vi "Priority system.vi"(0 "robot location":dbl[](array[numeric]), 1 "robot direction":string, 3 "Display Map":dbl[][](array[numeric])) -> (7 "Map":u16[][](array[ring]), 8 "target location":dbl[](array[numeric]))   [LabVIEW 2015]
uses:
  <vilib>/robotics/Navigation/shared/WorldMap/OccupancyGridWorldMap/NI_Robotics_OccupancyGridWorldMap.lvclass
  <vilib>/robotics/Navigation/NI_Robotics_Navigation .lvlib
panel:
  out "route map":dbl[][](array[numeric])
  out "distances":dbl[](array[numeric])
  out "Indices":i32[][](array[numeric])
  out "Priority level array":dbl[][](array[numeric])
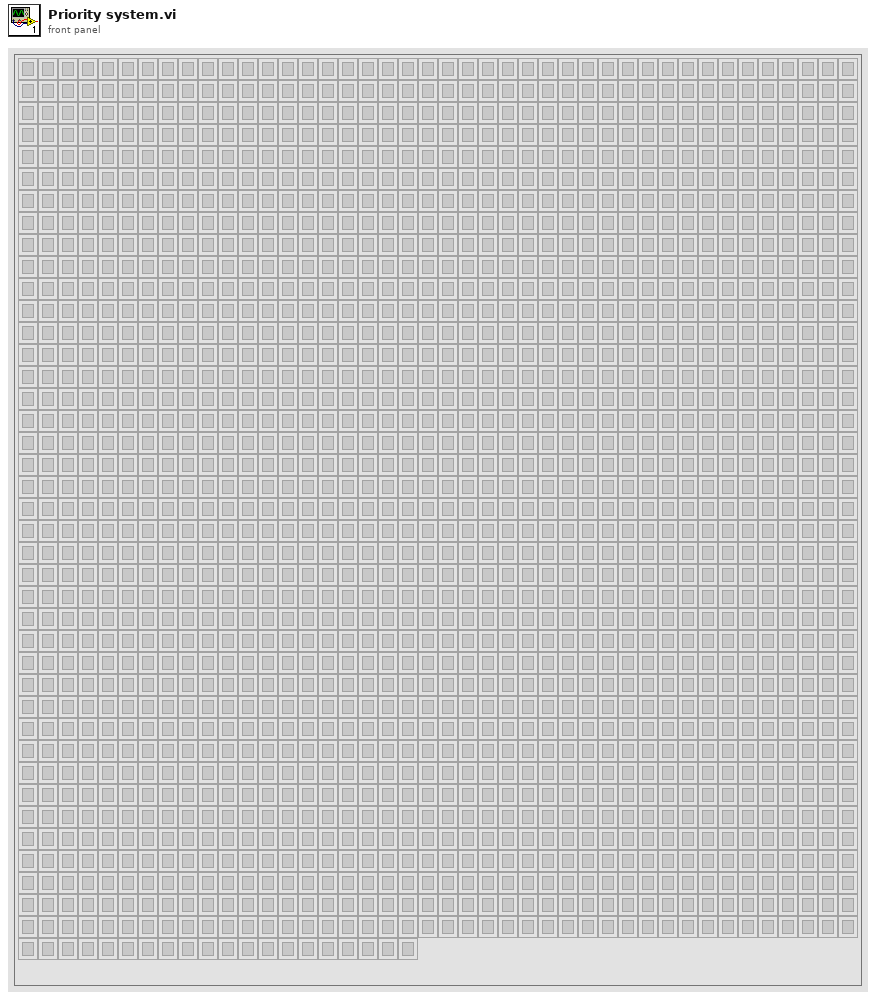
[diagram p1: front panel]
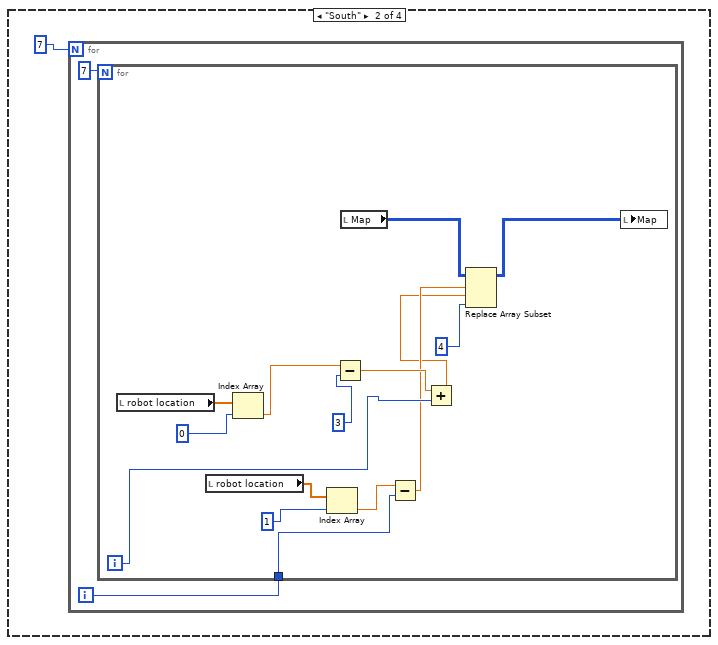
[diagram p2: hidden frame]
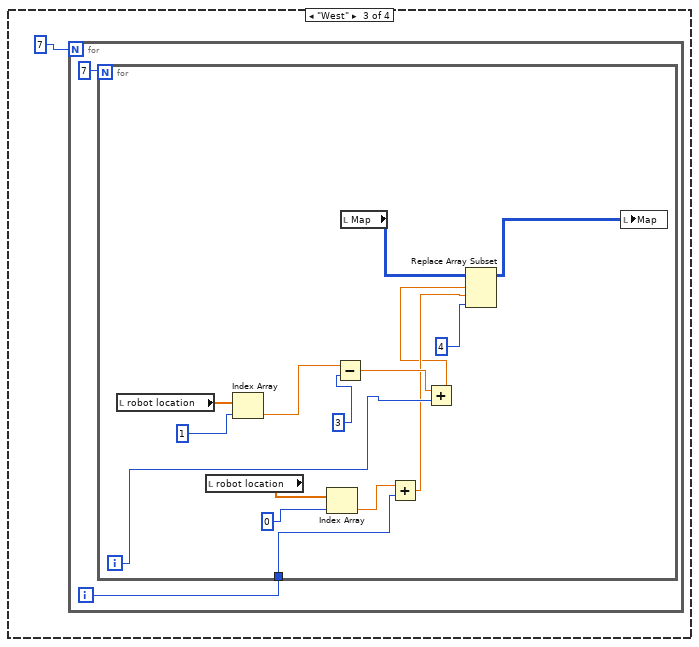
[diagram p3: hidden frame]
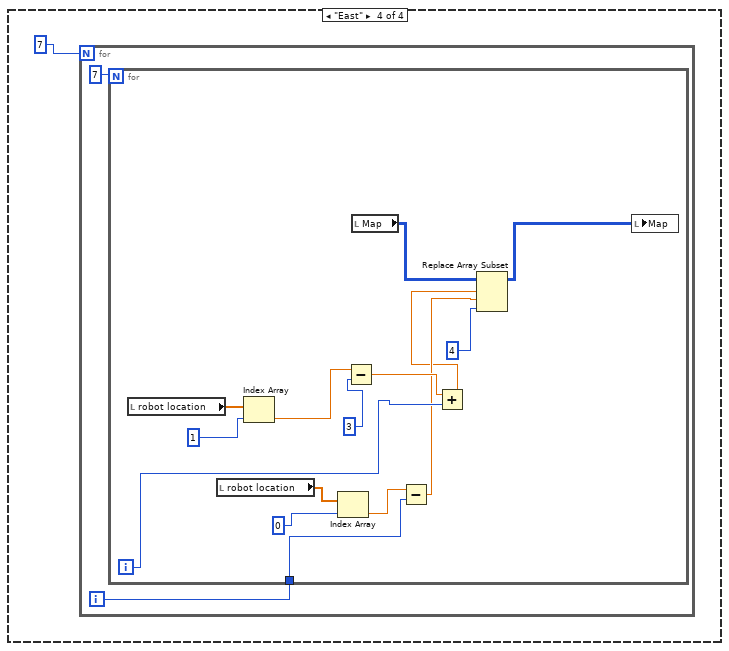
[diagram p4: hidden frame]
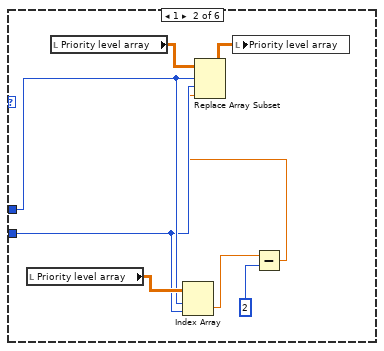
[diagram p6: hidden frame]
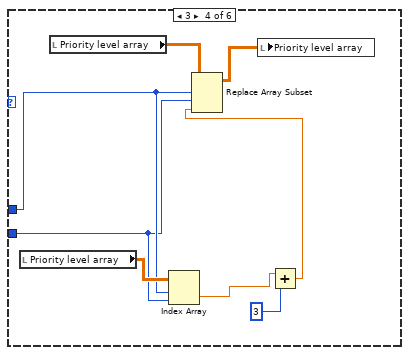
[diagram p8: hidden frame]
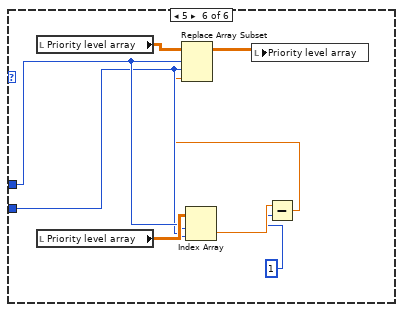
[diagram p9: hidden frame]
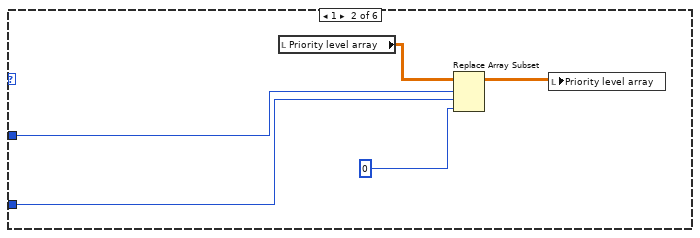
[diagram p10: hidden frame]
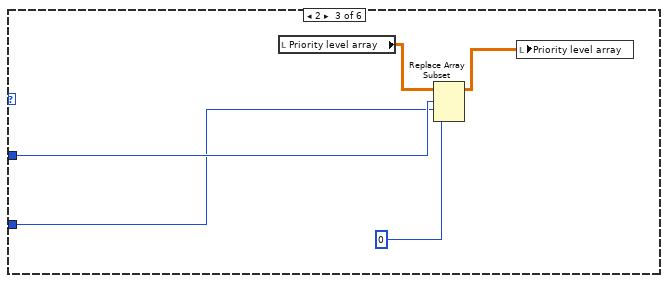
[diagram p11: hidden frame]
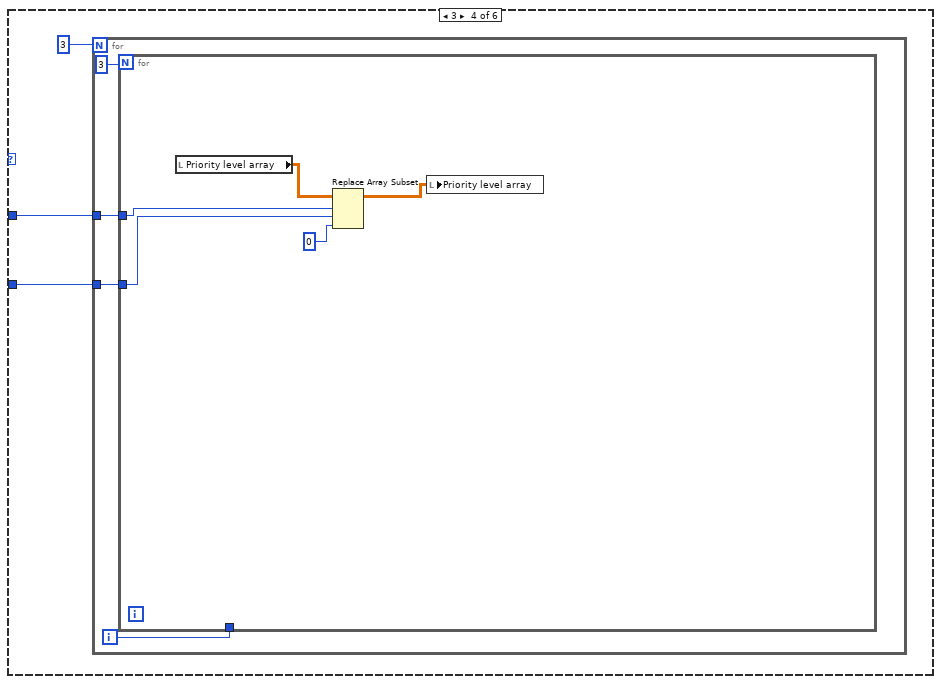
[diagram p12: hidden frame]
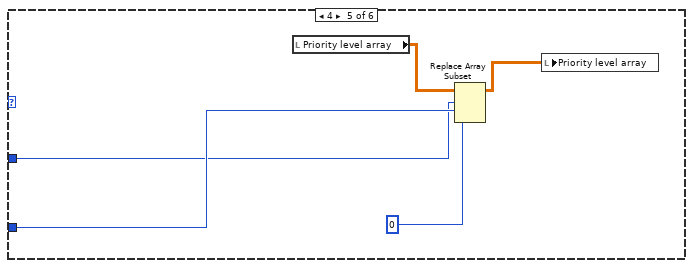
[diagram p13: hidden frame]
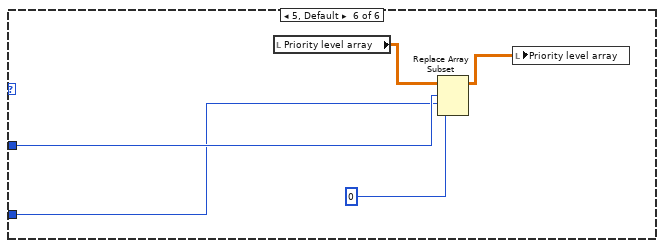
[diagram p14: hidden frame]
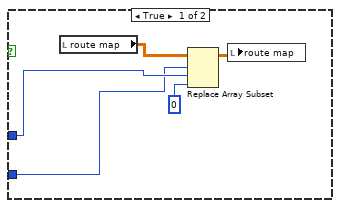
[diagram p16: hidden frame]
diagram:
  n1 = flat-sequence {
    frame #0 {
      "Map" <- "Display Map"
      "Priority level array" <- "Display Map"
      "route map" <- "Display Map"
    }
    frame #1 {
      n2 = for {
        N: 40 -> [_]
        i -> [w3]
        n3 = for {
          N: 40 -> [_]
          tunnel: w3 -> [w9]
          i -> [w10]
          n4 = local read "Priority level array"() -> (w5:dbl[][])
          n5 = local read "route map"() -> (w6:dbl[][])
          n6 = Replace Array Subset(array=w6, new element=0, index (row)=w10, index (col)=w9) -> (w11:dbl[][])
          n7 = Replace Array Subset(array=w5, new element=15, index (row)=w10, index (col)=w9) -> (w12:dbl[][])
          n8 = local write "Priority level array"(w12) -> ()
          n9 = local write "route map"(w11) -> ()
        }
      }
    }
    frame #2 {
      n10 = case shown="\"North\", Default" "robot direction" {
        frame "North", Default {
          n11 = for {
            N: 7 -> [_]
            i -> [w15]
            n12 = for {
              N: 7 -> [_]
              tunnel: w15 -> [w23]
              i -> [w27]
              n13 = local read "robot location"() -> (w17:dbl[])
              n14 = local read "robot location"() -> (w20:dbl[])
              n15 = Index Array(array=w17, index=0) -> (element=w18:dbl)
              n16 = Index Array(array=w20, index=1) -> (element=w19:dbl)
              n17 = Subtract(x=w18, y=3) -> (x-y=w26:dbl)
              n18 = local read "Map"() -> (w22:u16[][])
              n19 = Add(x=w19, y=w23) -> (x+y=w25:dbl)
              n20 = Add(x=w26, y=w27) -> (x+y=w24:dbl)
              n21 = Replace Array Subset(array=w22, new element=4, index (row)=w25, index (col)=w24) -> (w21:u16[][])
              n22 = local write "Map"(w21) -> ()
            }
          }
        }
        frame "South" {
          n23 = for {
            N: 7 -> [_]
            i -> [w33]
            n24 = for {
              N: 7 -> [_]
              tunnel: w33 -> [w41]
              i -> [w45]
              n25 = local read "robot location"() -> (w38:dbl[])
              n26 = local read "robot location"() -> (w37:dbl[])
              n27 = Index Array(array=w38, index=0) -> (element=w36:dbl)
              n28 = Index Array(array=w37, index=1) -> (element=w35:dbl)
              n29 = Subtract(x=w36, y=3) -> (x-y=w44:dbl)
              n30 = local read "Map"() -> (w40:u16[][])
              n31 = Subtract(x=w35, y=w41) -> (x-y=w43:dbl)
              n32 = Add(x=w44, y=w45) -> (x+y=w42:dbl)
              n33 = Replace Array Subset(array=w40, new element=4, index (row)=w43, index (col)=w42) -> (w39:u16[][])
              n34 = local write "Map"(w39) -> ()
            }
          }
        }
        frame "West" {
          n35 = for {
            N: 7 -> [_]
            i -> [w51]
            n36 = for {
              N: 7 -> [_]
              tunnel: w51 -> [w61]
              i -> [w63]
              n37 = local read "robot location"() -> (w56:dbl[])
              n38 = local read "robot location"() -> (w55:dbl[])
              n39 = Index Array(array=w56, index=1) -> (element=w54:dbl)
              n40 = Index Array(array=w55, index=0) -> (element=w53:dbl)
              n41 = Subtract(x=w54, y=3) -> (x-y=w62:dbl)
              n42 = local read "Map"() -> (w58:u16[][])
              n43 = Add(x=w53, y=w61) -> (x+y=w60:dbl)
              n44 = Add(x=w62, y=w63) -> (x+y=w59:dbl)
              n45 = Replace Array Subset(array=w58, new element=4, index (row)=w59, index (col)=w60) -> (w57:u16[][])
              n46 = local write "Map"(w57) -> ()
            }
          }
        }
        frame "East" {
          n47 = for {
            N: 7 -> [_]
            i -> [w69]
            n48 = for {
              N: 7 -> [_]
              tunnel: w69 -> [w73]
              i -> [w75]
              n49 = local read "robot location"() -> (w82:dbl[])
              n50 = local read "robot location"() -> (w80:dbl[])
              n51 = Index Array(array=w82, index=1) -> (element=w77:dbl)
              n52 = Index Array(array=w80, index=0) -> (element=w78:dbl)
              n53 = Subtract(x=w77, y=3) -> (x-y=w74:dbl)
              n54 = local read "Map"() -> (w85:u16[][])
              n55 = Subtract(x=w78, y=w73) -> (x-y=w72:dbl)
              n56 = Add(x=w74, y=w75) -> (x+y=w71:dbl)
              n57 = Replace Array Subset(array=w85, new element=4, index (row)=w71, index (col)=w72) -> (w84:u16[][])
              n58 = local write "Map"(w84) -> ()
            }
          }
        }
      }
    }
    frame #3 {
    }
    frame #4 {
      n59 = for {
        N: 40 -> [_]
        i -> [w87]
        n60 = for {
          N: 40 -> [_]
          tunnel: w87 -> [w91]
          i -> [w90]
          n61 = local read "Map"() -> (w92:u16[][])
          n62 = Index Array(array=w92, index (row)=w90, index (col)=w91) -> (element=w89:u16)
          n63 = case shown="0" w89 {
            tunnel: w91 -> [w95 w145 w151 w156 w168 w172]
            tunnel: w90 -> [w94 w144 w152 w155 w167 w173]
            frame 0 {
              n64 = for {
                N: 3 -> [_]
                tunnel: w95 -> [w99]
                tunnel: w94 -> [w98]
                i -> [w96]
                n65 = for {
                  N: 3 -> [_]
                  tunnel: w99 -> [w108]
                  tunnel: w98 -> [w107]
                  tunnel: w96 -> [w103]
                  i -> [w105]
                  n66 = Add(x=w107, y=1) -> (x+y=w106:i32)
                  n67 = Add(x=w108, y=1) -> (x+y=w104:i32)
                  n68 = local read "Map"() -> (w111:u16[][])
                  n69 = Subtract(x=w106, y=w105) -> (x-y=w101:i32)
                  n70 = Subtract(x=w104, y=w103) -> (x-y=w102:i32)
                  n71 = Index Array(array=w111, index (row)=w101, index (col)=w102) -> (element=w100:u16)
                  n72 = case shown="4" w100 {
                    tunnel: w108 -> [_ w115 _ w124 w131 w139]
                    tunnel: w107 -> [_ w116 _ w125 w132 w140]
                    frame 0, Default {
                    }
                    frame 1 {
                      n73 = local read "Priority level array"() -> (w119:dbl[][])
                      n74 = local read "Priority level array"() -> (w118:dbl[][])
                      n75 = Index Array(array=w119, index (row)=w116, index (col)=w115) -> (element=w114:dbl)
                      n76 = Subtract(x=w114, y=2) -> (x-y=w112:dbl)
                      n77 = Replace Array Subset(array=w118, new element=w112, index (row)=w116, index (col)=w115) -> (w117:dbl[][])
                      n78 = local write "Priority level array"(w117) -> ()
                    }
                    frame 2 {
                    }
                    frame 3 {
                      n79 = local read "Priority level array"() -> (w126:dbl[][])
                      n80 = local read "Priority level array"() -> (w127:dbl[][])
                      n81 = Index Array(array=w126, index (row)=w125, index (col)=w124) -> (element=w123:dbl)
                      n82 = Add(x=w123, y=3) -> (x+y=w121:dbl)
                      n83 = Replace Array Subset(array=w127, new element=w121, index (row)=w125, index (col)=w124) -> (w122:dbl[][])
                      n84 = local write "Priority level array"(w122) -> ()
                    }
                    frame 4 {
                      n85 = local read "Priority level array"() -> (w133:dbl[][])
                      n86 = local read "Priority level array"() -> (w135:dbl[][])
                      n87 = Index Array(array=w133, index (row)=w132, index (col)=w131) -> (element=w130:dbl)
                      n88 = Subtract(x=w130, y=0) -> (x-y=w129:dbl)
                      n89 = Replace Array Subset(array=w135, new element=w129, index (row)=w132, index (col)=w131) -> (w134:dbl[][])
                      n90 = local write "Priority level array"(w134) -> ()
                    }
                    frame 5 {
                      n91 = local read "Priority level array"() -> (w141:dbl[][])
                      n92 = local read "Priority level array"() -> (w143:dbl[][])
                      n93 = Index Array(array=w143, index (row)=w140, index (col)=w139) -> (element=w138:dbl)
                      n94 = Subtract(x=w138, y=1) -> (x-y=w137:dbl)
                      n95 = Replace Array Subset(array=w141, new element=w137, index (row)=w140, index (col)=w139) -> (w142:dbl[][])
                      n96 = local write "Priority level array"(w142) -> ()
                    }
                  }
                }
              }
            }
            frame 1 {
              n97 = local read "Priority level array"() -> (w148:dbl[][])
              n98 = Replace Array Subset(array=w148, new element=0, index (row)=w144, index (col)=w145) -> (w147:dbl[][])
              n99 = local write "Priority level array"(w147) -> ()
            }
            frame 2 {
              n100 = local read "Priority level array"() -> (w153:dbl[][])
              n101 = Replace Array Subset(array=w153, new element=0, index (row)=w152, index (col)=w151) -> (w150:dbl[][])
              n102 = local write "Priority level array"(w150) -> ()
            }
            frame 3 {
              n103 = for {
                N: 3 -> [_]
                tunnel: w156 -> [w160]
                tunnel: w155 -> [w159]
                i -> [w157]
                n104 = for {
                  N: 3 -> [_]
                  tunnel: w160 -> [w161]
                  tunnel: w159 -> [w162]
                  tunnel: w157 -> [_]
                  n105 = local read "Priority level array"() -> (w165:dbl[][])
                  n106 = Replace Array Subset(array=w165, new element=0, index (row)=w162, index (col)=w161) -> (w164:dbl[][])
                  n107 = local write "Priority level array"(w164) -> ()
                }
              }
            }
            frame 4 {
              n108 = local read "Priority level array"() -> (w170:dbl[][])
              n109 = Replace Array Subset(array=w170, new element=0, index (row)=w167, index (col)=w168) -> (w169:dbl[][])
              n110 = local write "Priority level array"(w169) -> ()
            }
            frame 5, Default {
              n111 = local read "Priority level array"() -> (w175:dbl[][])
              n112 = Replace Array Subset(array=w175, new element=0, index (row)=w173, index (col)=w172) -> (w174:dbl[][])
              n113 = local write "Priority level array"(w174) -> ()
            }
          }
        }
      }
    }
    frame #5 {
      n114 = local read "Priority level array"() -> (w177:dbl[][])
      n115 = for {
        tunnel: [w180] -> _ mode=indexing
        shift-right: [w184] -> w179
        shift-left: i32[][] [] -> [w182]
        tunnel: w177 -> [w180] mode=indexing
        i -> [w186]
        n116 = Increment(x=w186) -> (x+1=w185:i32)
        n117 = for {
          tunnel: w180 -> [w195] mode=indexing
          tunnel: w185 -> [w191]
          shift-right: [w190] -> w183
          shift-left: i32[][] [] -> [w189]
          i -> [w193]
          n118 = local read "Priority level array"() -> (w188:dbl[][])
          n119 = Array Max & Min(array=w188) -> (max value=w187:dbl)  [unwired: 3 out]
          n120 = Equal?(x=w195, y=w187) -> (x = y?=w194:bool)
          n121 = Increment(x=w193) -> (x+1=w192:i32)
          n122 = case shown="True" w194 {
            tunnel: w192 -> [_ w201]
            tunnel: w191 -> [_ w200]
            tunnel: [w196 w198] -> w190
            tunnel: w189 -> [w196 w197]
            frame False {
            }
            frame True {
              n123 = Build Array(w201, w200) -> (w199:i32[])
              n124 = Build Array (concatenate)(w197, w199) -> (w198:i32[][])
            }
          }
        }
        n125 = Build Array (concatenate)(w182, w183) -> (w184:i32[][])
      }
      "Indices" <- w179
      "distances" <- i32[] [0, 0, 0, 0]
    }
    frame #6 {
      n126 = for {
        N: 10 -> [_]
        i -> [w204]
        n127 = local read "Indices"() -> (w226:i32[][])
        n128 = Index Array(array=w226, index (row)=w204, index (col)=0) -> (element=w218:i32)
        n129 = Index Array(array=w226, index (row)=w204, index (col)=1) -> (element=w217:i32)
        n130 = Index Array(array="robot location", index=1) -> (element=w220:dbl)
        n131 = Index Array(array="robot location", index=0) -> (element=w222:dbl)
        n132 = Add(x=w220, y=1) -> (x+y=w215:dbl)
        n133 = Add(x=w222, y=1) -> (x+y=w216:dbl)
        n134 = Subtract(x=w218, y=w216) -> (x-y=w214:dbl)
        n135 = Subtract(x=w217, y=w215) -> (x-y=w207:dbl)
        n136 = Square(x=w207) -> (x^2=w213:dbl)
        n137 = Square(x=w214) -> (x^2=w212:dbl)
        n138 = Add(x=w212, y=w213) -> (x+y=w211:dbl)
        n139 = local read "distances"() -> (w210:dbl[])
        n140 = Square Root(x=w211) -> (sqrt(x)=w208:dbl)
        n141 = Replace Array Subset(array=w210, new element=w208, index=w204) -> (w209:dbl[])
        n142 = local write "distances"(w209) -> ()
      }
      "target location" <- i32[] [0, 0]
    }
    frame #7 {
      n143 = local read "distances"() -> (w234:dbl[])
      n144 = local read "Indices"() -> (w227:i32[][])
      n145 = Array Max & Min(array=w234) -> (min index (indices)=w229:i32)  [unwired: 3 out]
      n146 = local read "target location"() -> (w231:dbl[])
      n147 = Index Array(array=w227, index (row)=w229, index (col)=0) -> (element=w232:i32)
      n148 = Replace Array Subset(array=w231, new element=w232, index=0) -> (w233:dbl[])
      n149 = local write "target location"(w233) -> ()
    }
    frame #8 {
      n150 = local read "distances"() -> (w241:dbl[])
      n151 = local read "Indices"() -> (w240:i32[][])
      n152 = Array Max & Min(array=w241) -> (min index (indices)=w242:i32)  [unwired: 3 out]
      n153 = local read "target location"() -> (w237:dbl[])
      n154 = Index Array(array=w240, index (row)=w242, index (col)=1) -> (element=w236:i32)
      n155 = Replace Array Subset(array=w237, new element=w236, index=1) -> (w235:dbl[])
      n156 = local write "target location"(w235) -> ()
    }
    frame #9 {
      n157 = local read "target location"() -> (w249:dbl[])
      n158 = Index Array(array=w249, index #1=0, index #2=1) -> (element #1=w246:dbl, element #2=w245:dbl)
      n159 = local read "Map"() -> (w252:u16[][])
      n160 = Decrement(x=w245) -> (x-1=w244:dbl)
      n161 = Decrement(x=w246) -> (x-1=w243:dbl)
      n162 = Replace Array Subset(array=w252, new element=4, index (row)=w244, index (col)=w243) -> (w251:u16[][])
      n163 = local write "Map"(w251) -> ()
    }
    frame #10 {
      n164 = for {
        N: 40 -> [_]
        i -> [w254]
        n165 = for {
          N: 40 -> [_]
          tunnel: w254 -> [w259]
          i -> [w260]
          n166 = local read "Priority level array"() -> (w261:dbl[][])
          n167 = Index Array(array=w261, index (row)=w260, index (col)=w259) -> (element=w257:dbl)
          n168 = Equal?(x=w257, y=15) -> (x = y?=w258:bool)
          n169 = case shown="False" w258 {
            tunnel: w260 -> [w262 w268]
            tunnel: w259 -> [w263 w267]
            frame True {
              n170 = local read "route map"() -> (w265:dbl[][])
              n171 = Replace Array Subset(array=w265, new element=0, index (row)=w262, index (col)=w263) -> (w266:dbl[][])
              n172 = local write "route map"(w266) -> ()
            }
            frame False {
              n173 = local read "route map"() -> (w270:dbl[][])
              n174 = Replace Array Subset(array=w270, new element=1, index (row)=w268, index (col)=w267) -> (w269:dbl[][])
              n175 = local write "route map"(w269) -> ()
            }
          }
        }
      }
    }
    frame #11 {
      n176 = local read "route map"() -> (w284:dbl[][])
      n177 = local read "robot location"() -> (w283:dbl[])
      n178 = Multiply(x=w284, y=99) -> (x*y=w295:dbl[][])
      n179 = Add(x=w295, y=1) -> (x+y=w293:dbl[][])
      n180 = call <vilib>:"Create Occupancy Grid Map.vi"("occupancy grid"=w293) -> ("error out"=w292:errorcluster, "map reference out"=w288:refnum<data-value>)  [unwired: 9 in]
      n181 = Index Array(array=w283, index #1=0, index #2=1) -> (element #1=w273:dbl, element #2=w272:dbl)
      n182 = local read "target location"() -> (w280:dbl[])
      n183 = call <vilib>:"Get Cell Reference.vi"("error in (no error)"=w292, "y"=w273, "x"=w272, "map reference in"=w288) -> ("error out"=w291:errorcluster, "cell reference"=w289:refnum<data-value>, "map reference out"=w301:refnum<data-value>)  [unwired: 4 in, 1 out]
      n184 = Index Array(array=w280, index #1=0, index #2=1) -> (element #1=w277:dbl, element #2=w276:dbl)
      n185 = Decrement(x=w276) -> (x-1=w274:dbl)
      n186 = Decrement(x=w277) -> (x-1=w275:dbl)
      n187 = call <vilib>:"Get Cell Reference.vi"("error in (no error)"=w291, "y"=w275, "x"=w274, "map reference in"=w301) -> ("error out"=w290:errorcluster, "cell reference"=w287:refnum<data-value>, "map reference out"=w299:refnum<data-value>)  [unwired: 4 in, 1 out]
      n188 = call <vilib>:"A Star Plan.vi"("goal reference"=w287, "start reference"=w289, "map reference in"=w299) -> ("path references"=w300:refnum<data-value>[])  [unwired: 5 in, 3 out]
      n189 = call <vilib>:"Get Cells in Path.vi"("error in (no error)"=w290, "path references"=w300, "map reference in"=w299) -> ("error out"=w285:errorcluster, "y coordinates"=w298:i32[], "x coordinates"=w297:i32[], "map reference out"=w286:refnum<data-value>)  [unwired: 5 in]
      n190 = for {
        tunnel: w298 -> [w305] mode=indexing
        tunnel: w297 -> [w306] mode=indexing
        n191 = local read "Map"() -> (w302:u16[][])
        n192 = Replace Array Subset(array=w302, new element=2, index (row)=w306, index (col)=w305) -> (w303:u16[][])
        n193 = local write "Map"(w303) -> ()
      }
      n194 = call <vilib>:"Close Occupancy Grid Map.vi"("error in (no error)"=w285, "map reference in"=w286) -> ()  [unwired: 9 in, 1 out]
    }
    frame #12 {
      n195 = local read "robot location"() -> (w309:dbl[])
      n196 = local read "robot location"() -> (w310:dbl[])
      n197 = local read "Map"() -> (w311:u16[][])
      n198 = Index Array(array=w309, index=0) -> (element=w308:dbl)
      n199 = Index Array(array=w310, index=1) -> (element=w313:dbl)
      n200 = Replace Array Subset(array=w311, new element=5, index (row)=w313, index (col)=w308) -> (w312:u16[][])
      n201 = local write "Map"(w312) -> ()
    }
  }
